vi "Keithley 2450 Read Multiple.vi"() -> ()   [LabVIEW 2021]
doc: "This example shows how to configure a measurement and take multiple readings."
uses:
  <instrlib>/Keithley 2450/Keithley 2450.lvlib
panel:
  in  "Compliance Level (0.1)":dbl=0.1
  in  "Output Level (0)":dbl
  in  "Source Mode  (0: Voltage)":u16(ring) items=["Voltage", "Current"]
  out "Resistance":sgl[](array[numeric])
  out "Current":sgl[](array[numeric])
  out "Voltage":sgl[](array[numeric])
  in  "VISA resource name":refnum<visa-resource-name>
  # "(c) 2021 National Instruments.  ALL RIGHTS RESERVED."
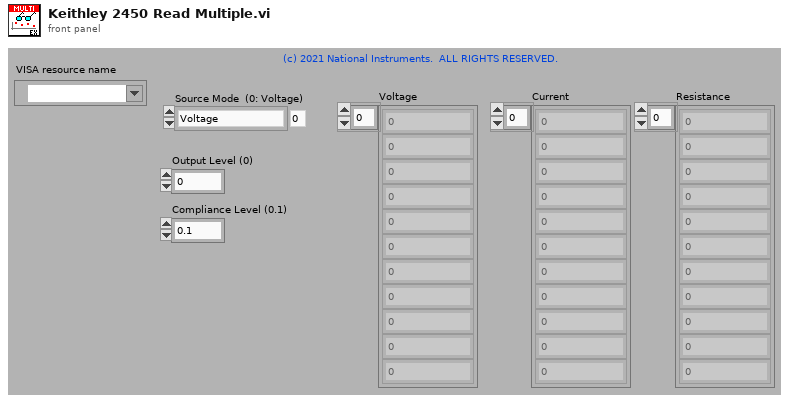
[diagram p1: front panel]
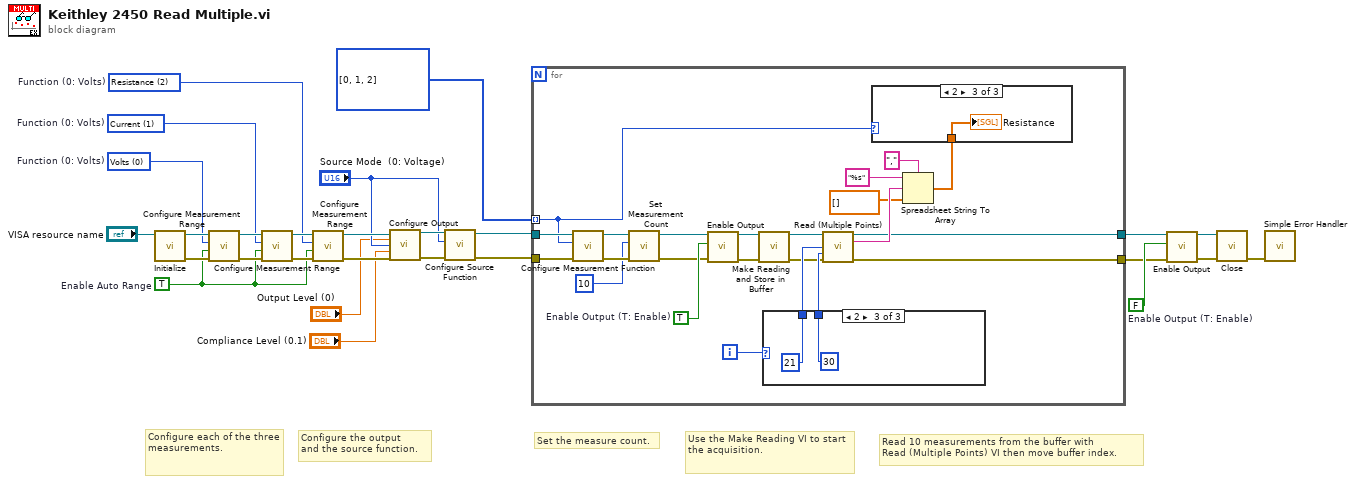
[diagram p0: block diagram]
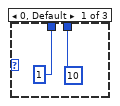
[diagram p2: hidden frame]
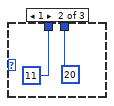
[diagram p3: hidden frame]
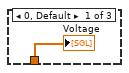
[diagram p4: hidden frame]
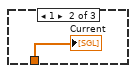
[diagram p5: hidden frame]
diagram:
  w8 = u16[] [0, 1, 2] items=["Volts", "Current", "Resistance"]
  w13 = FALSE  # Enable Output (T: Enable)
  w16 = u16 2 items=["Volts", "Current", "Resistance"]  # Function (0: Volts)
  w17 = u16 1 items=["Volts", "Current", "Resistance"]  # Function (0: Volts)
  w18 = u16 0 items=["Volts", "Current", "Resistance"]  # Function (0: Volts)
  w19 = TRUE  # Enable Auto Range
  # "Read 10 measurements from the buffer with \nRead (Multiple Points) VI then move buffer index."
  # "Set the measure count."
  # "Use the Make Reading VI to start the acquisition."
  # "Configure the output \nand the source function."
  # "Configure each of the three measurements."
  n1 = call <instrlib>:"Initialize.vi"("VISA resource name"="VISA resource name") -> ("error out"=w24:errorcluster, "VISA resource name out"=w25:refnum<visa-resource-name>)  [unwired: 9 in]
  n2 = call <instrlib>:"Configure Measurement Range.vi"("error in (no error)"=w24, "Enable Auto Range (T:Enable)"=w19, "Function (0: Volts)"=w18, "VISA resource name"=w25) -> ("error out"=w23:errorcluster, "VISA resource name out"=w22:refnum<visa-resource-name>)  [unwired: 6 in]
  n3 = call <instrlib>:"Configure Measurement Range.vi"("error in (no error)"=w23, "Enable Auto Range (T:Enable)"=w19, "Function (0: Volts)"=w17, "VISA resource name"=w22) -> ("error out"=w20:errorcluster, "VISA resource name out"=w21:refnum<visa-resource-name>)  [unwired: 6 in]
  n4 = call <instrlib>:"Configure Measurement Range.vi"("error in (no error)"=w20, "Enable Auto Range (T:Enable)"=w19, "Function (0: Volts)"=w16, "VISA resource name"=w21) -> ("error out"=w11:errorcluster, "VISA resource name out"=w12:refnum<visa-resource-name>)  [unwired: 6 in]
  n5 = call <instrlib>:"Configure Output.vi"("VISA resource name"=w12, "Source Level (0)"="Output Level (0)", "Source Mode  (0: Voltage)"="Source Mode  (0: Voltage)", "Source Limit Level (0.1)"="Compliance Level (0.1)", "error in (no error)"=w11) -> ("VISA resource name out"=w6:refnum<visa-resource-name>, "error out"=w7:errorcluster)  [unwired: 9 in]
  n6 = call <instrlib>:"Configure Source Function.vi"("error in (no error)"=w7, "Function (0: Volts)"="Source Mode  (0: Voltage)", "VISA resource name"=w6) -> ("error out"=w4:errorcluster, "VISA resource name out"=w5:refnum<visa-resource-name>)  [unwired: 7 in]
  n7 = for {
    tunnel: [w39] -> w10
    tunnel: [w38] -> w9
    tunnel: w4 -> [w50]
    tunnel: w5 -> [w49]
    tunnel: w8 -> [w48] mode=indexing
    i -> [w35]
    w32 = TRUE  # Enable Output (T: Enable)
    n8 = call <instrlib>:"Configure Measurement Function.vi"("error in (no error)"=w50, "Function (0: Volts)"=w48, "VISA resource name"=w49) -> ("error out"=w47:errorcluster, "VISA resource name out"=w46:refnum<visa-resource-name>)  [unwired: 7 in]
    n9 = call <instrlib>:"Set Measurement Count.vi"("error in (no error)"=w47, "Measurement Count (1)"=u32 10 ("millisecond multiple"), "VISA resource name"=w46) -> ("error out"=w30:errorcluster, "VISA resource name out"=w31:refnum<visa-resource-name>)  [unwired: 7 in]
    n10 = call <instrlib>:"Enable Output.vi"("error in (no error)"=w30, "Enable Output (T: Enable)"=w32, "VISA resource name"=w31) -> ("error out"=w28:errorcluster, "VISA resource name out"=w29:refnum<visa-resource-name>)  [unwired: 7 in]
    n11 = call <instrlib>:"Make Reading and Store in Buffer.vi"("VISA resource name"=w29, "error in (no error)"=w28) -> ("VISA resource name out"=w34:refnum<visa-resource-name>, "error out"=w33:errorcluster)  [unwired: 12 in]
    n12 = case shown="2" w35 {
      tunnel: [u32 1 ("millisecond multiple") u32 11 ("millisecond multiple") u32 21 ("millisecond multiple")] -> w37
      tunnel: [u32 10 ("millisecond multiple") u32 20 ("millisecond multiple") u32 30 ("millisecond multiple")] -> w36
      frame 0, Default {
      }
      frame 1 {
      }
      frame 2 {
      }
    }
    n13 = call <instrlib>:"Read (Multiple Points).vi"("VISA resource name"=w34, "Start Index (1)"=w37, "End Index (1)"=w36, "error in (no error)"=w33) -> ("VISA resource name out"=w39:refnum<visa-resource-name>, "Data out"=w44:string, "error out"=w38:errorcluster)  [unwired: 9 in]
    n14 = Spreadsheet String To Array(delimiter (Tab)=",", format string="%s", spreadsheet string=w44, array type (2D Dbl)=dbl[] []) -> (array=w43:dbl[])
    n15 = case shown="2" w48 {
      tunnel: w43 -> [w57 w58 w59]
      frame 0, Default {
        "Voltage" <- w57
      }
      frame 1 {
        "Current" <- w58
      }
      frame 2 {
        "Resistance" <- w59
      }
    }
  }
  n16 = call <instrlib>:"Enable Output.vi"("error in (no error)"=w9, "Enable Output (T: Enable)"=w13, "VISA resource name"=w10) -> ("error out"=w14:errorcluster, "VISA resource name out"=w15:refnum<visa-resource-name>)  [unwired: 7 in]
  n17 = call <instrlib>:"Close.vi"("error in (no error)"=w14, "VISA resource name"=w15) -> ("error out"=w27:errorcluster)  [unwired: 9 in]
  n18 = call <vilib>:"Simple Error Handler.vi"("error in (no error)"=w27) -> ()  [unwired: 4 in, 5 out]
